vi "calcCompensatorOutput.vi"(6 "reinitializeIsTrue":bool, 8 "error in (no error)":errorcluster, 9 "Force Measured":T2 min=-888.0 max=888.0 format="%.2f", 10 "Force Setpoint":T2 min=-888.0 max=888.0 format="%.2f", 11 "PressureTransducerCompensator in":refnum<class "PressureTransducerCompensator.lvclass">) -> (0 "error out":errorcluster, 2 "Pressure Transducer Setpoint":T1 {"Tension" min=-888.0 max=888.0 format="%.2f"; "Compression" min=-888.0 max=888.0 format="%.2f"}, 3 "PressureTransducerCompensator out":refnum<class "PressureTransducerCompensator.lvclass">)   [LabVIEW 2013, in "PressureTransducerCompensator.lvclass"]
uses:
  PressureTransducerCompensator.lvclass
  Typedefs/ForceSetpoint.ctl
  Typedefs/PressureTransducerSetpoint.ctl
  PressureTransducerCompensator.lvclass/PressureTransducerCompensator.ctl
  <vilib>/addons/control/pid/NI_PID_pid.lvlib
  Typedefs/FAMTTypedefs.lvlib
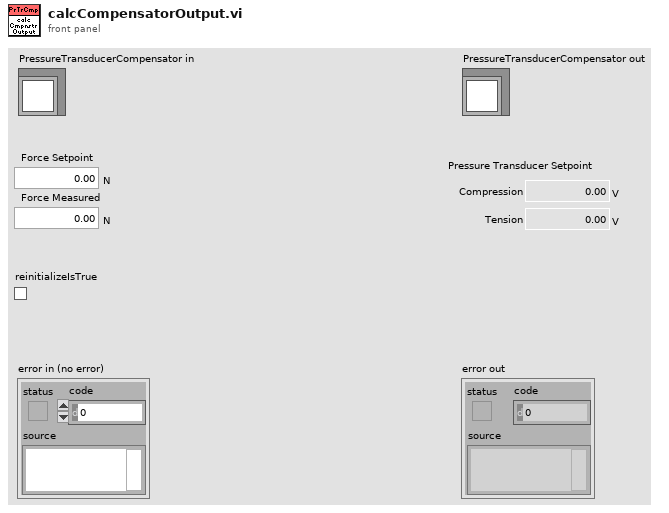
[diagram p1: front panel]
types:
  T1 = typedef "FAMTTypedefs.lvlib/PressureTransducerSetpoint.ctl" = cluster{"Compression":dbl[unit], "Tension":dbl[unit]}
  T2 = typedef "FAMTTypedefs.lvlib/ForceSetpoint.ctl" = dbl[unit]
  T3 = typedef "PIDGains.ctl" = cluster{"Proportional Gain (Kc)":dbl, "Integral Time (Ti, min)":dbl, "Derivative Time (Td, min)":dbl}
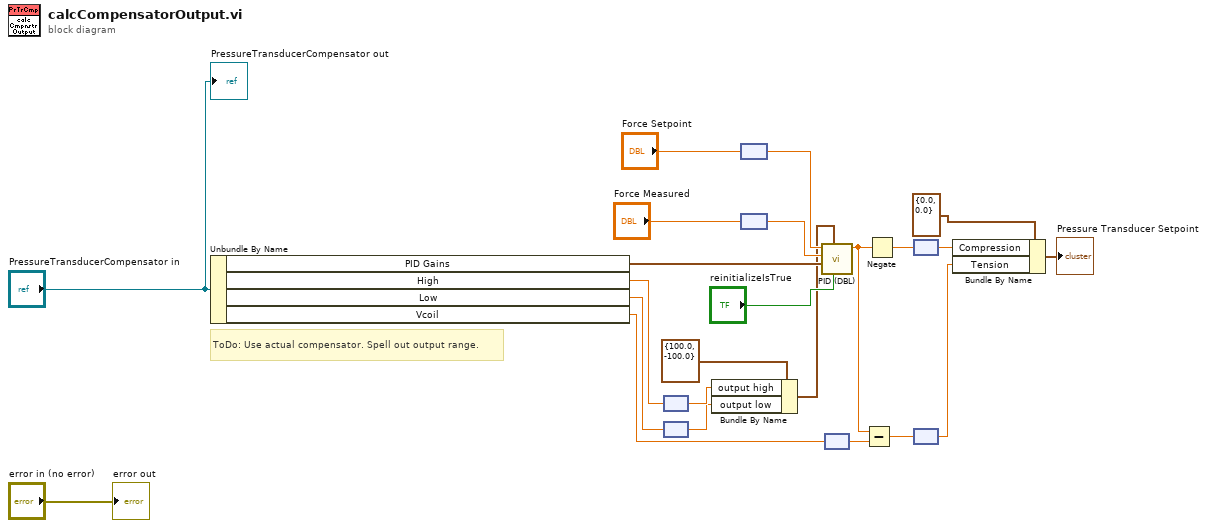
[diagram p0: block diagram]
diagram:
  # "ToDo: Use actual compensator. Spell out output range."
  n1 = Unbundle By Name("PressureTransducerCompensator in") -> ("PID Gains"=w7:T3, "High"=w6:dbl[unit], "Low"=w2:dbl[unit], "Vcoil"=w12:dbl[unit])
  n2 = node(w6) -> (w3:dbl)
  n3 = node(w2) -> (w1:dbl)
  n4 = Bundle By Name(cluster=cluster{"output high":dbl, "output low":dbl} {"output high"=100.0, "output low"=-100.0} ("output range"), "output high"=w3, "output low"=w1) -> (w4:cluster{"output high":dbl, "output low":dbl})
  n5 = node("Force Setpoint") -> (w18:dbl)
  n6 = node("Force Measured") -> (w19:dbl)
  n7 = call <vilib>:"PID (DBL).vi"("reinitialize? (F)"="reinitializeIsTrue", "output range"=w4, "PID gains"=w7, "process variable"=w19, "setpoint"=w18) -> ("output"=w13:dbl)  [unwired: 5 in, 1 out]
  n8 = node(w12) -> (w11:dbl)
  n9 = Subtract(x=w13, y=w11) -> (x-y=w10:dbl)
  n10 = Negate(x=w13) -> (-x=w15:dbl)
  n11 = node(w15) -> (w14:dbl[unit])
  n12 = node(w10) -> (w9:dbl[unit])
  n13 = Bundle By Name(cluster=T1 {"Compression"=0.0, "Tension"=0.0} ("Pressure Transducer Setpoint"), "Compression"=w14, "Tension"=w9) -> (→"Pressure Transducer Setpoint":T1)
  "error out" <- "error in (no error)"
  "PressureTransducerCompensator out" <- "PressureTransducerCompensator in"
